vi "getAngle.vi"(6 "Axis":T1, 8 "error in (no error)":errorcluster, 11 "Instrument.Cryostat in":refnum<class "Instrument.Cryostat.lvclass">) -> (0 "error out":errorcluster, 1 "Status":string, 2 "Angle (°)":dbl, 3 "Instrument.Cryostat out":refnum<class "Instrument.Cryostat.lvclass">)   [LabVIEW 2019, in "Instrument.Cryostat.lvclass"]
uses:
  Instrument.Cryostat.lvclass
  C:/Users/patrick/Documents/GitHub/Instrument-Framework/lvsrc/Instrument/Instrument.lvclass
  Typedefs/Rotator Axis--Enum.ctl
  Typedefs/getAngle--cluster.ctl
  Instrument/Instrument.lvclass/Instrument.ctl
  d7de1868-e79d-4787-9e9f-00102efb34a0.vi
  d7de1868-e79d-4787-9e9f-00102efb34a0.vi/29015152-4dd0-45c0-ae7b-e0ee80cdf932.vi
  d7de1868-e79d-4787-9e9f-00102efb34a0.vi/78c8e4cc-1710-4685-8e18-4a9f090162ba.vi
  Instrument/Private/Get Client Type.vi
  d7de1868-e79d-4787-9e9f-00102efb34a0.vi/29015152-4dd0-45c0-ae7b-e0ee80cdf932.vi/49513277-8b05-47b5-8656-0540af669f9a.vi
  d7de1868-e79d-4787-9e9f-00102efb34a0.vi/29015152-4dd0-45c0-ae7b-e0ee80cdf932.vi/bcc89b85-e935-4bd8-847f-6a809bd2d440.vi
  Instrument/Private/Set Dependencies.vi
  d7de1868-e79d-4787-9e9f-00102efb34a0.vi/78c8e4cc-1710-4685-8e18-4a9f090162ba.vi/8cbdd292-283f-4f32-a3cc-82cdd24e7583.vi
  d7de1868-e79d-4787-9e9f-00102efb34a0.vi/78c8e4cc-1710-4685-8e18-4a9f090162ba.vi/036cd682-c314-48e0-a153-600fb577c118.vi
  d7de1868-e79d-4787-9e9f-00102efb34a0.vi/78c8e4cc-1710-4685-8e18-4a9f090162ba.vi/5d11e547-53d6-4100-b73f-5ffdf814e87d.vi
  d7de1868-e79d-4787-9e9f-00102efb34a0.vi/29015152-4dd0-45c0-ae7b-e0ee80cdf932.vi/bcc89b85-e935-4bd8-847f-6a809bd2d440.vi/2e8ce9c0-d7f6-46c2-b56a-ccad562160a9.vi
  d7de1868-e79d-4787-9e9f-00102efb34a0.vi/29015152-4dd0-45c0-ae7b-e0ee80cdf932.vi/bcc89b85-e935-4bd8-847f-6a809bd2d440.vi/071ed579-4f01-4414-bbcb-77796d1fffd3.vi
  d7de1868-e79d-4787-9e9f-00102efb34a0.vi/78c8e4cc-1710-4685-8e18-4a9f090162ba.vi/036cd682-c314-48e0-a153-600fb577c118.vi/f30586f2-7be0-47a0-9240-ffa99525c1ce.vi
  d7de1868-e79d-4787-9e9f-00102efb34a0.vi/78c8e4cc-1710-4685-8e18-4a9f090162ba.vi/036cd682-c314-48e0-a153-600fb577c118.vi/7bb9839c-ec85-4b4c-931f-28db1f4f848b.vi
  d7de1868-e79d-4787-9e9f-00102efb34a0.vi/78c8e4cc-1710-4685-8e18-4a9f090162ba.vi/5d11e547-53d6-4100-b73f-5ffdf814e87d.vi/70780e69-106e-4e28-be9f-45ae0745826c.vi
  d7de1868-e79d-4787-9e9f-00102efb34a0.vi/78c8e4cc-1710-4685-8e18-4a9f090162ba.vi/5d11e547-53d6-4100-b73f-5ffdf814e87d.vi/f098dfd7-b95c-4643-8807-c1855e54edfe.vi
  Instrument/Private/Get RC Connection Status.vi
  Instrument/Private/Get Dependencies.vi
  <userlib>/LevyLab/RemoteControl/API/Send and Receive.vi
  <vilib>/Utility/Data Type/Get Type Information.vi
  <vilib>/JDP Science/JSONtext/JSON text to Variant.vi
  Instrument/API/Instrument.GetPublicEvents.vi
  <vilib>/JDP Science/JSONtext/Variant to JSON Text.vi
  <vilib>/National Instruments/GUID Generator/Guid Generator.vi
  Instrument/API/Instrument.sendMessageToProcess.vi
  Instrument/Private/Instrument.MessageFromProcess.EventStructure.vi
  <vilib>/JDP Science/JSONtext/LVClass Serializer/JSONtext LVClass Serializer.lvclass
  Instrument/Instrument.lvclass
panel:
  out "Finished?":bool
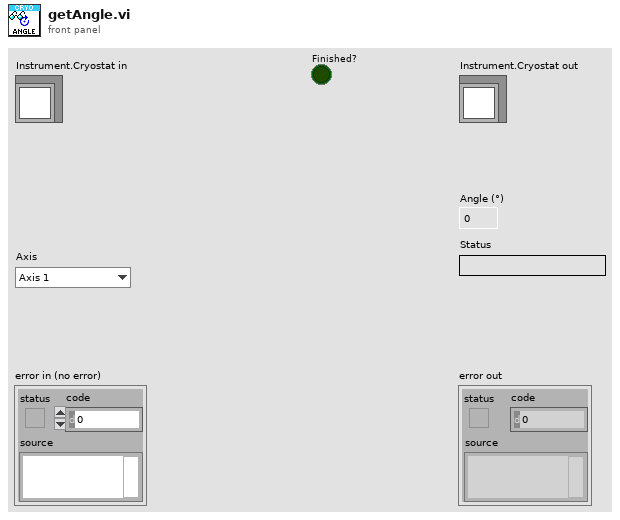
[diagram p1: front panel]
types:
  T1 = typedef "Instrument.Cryostat.lvclass/Rotator Axis--Enum.ctl" = enum16{"Axis 1", "Axis 2"}
  T2 = typedef "Instrument.Cryostat.lvclass/getAngle--cluster.ctl" = cluster{"Angle":dbl, "Status":string, "Finished?":bool}
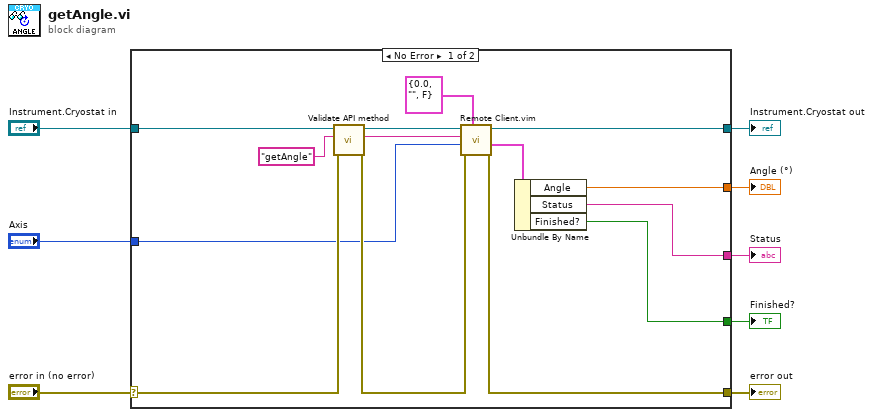
[diagram p0: block diagram]
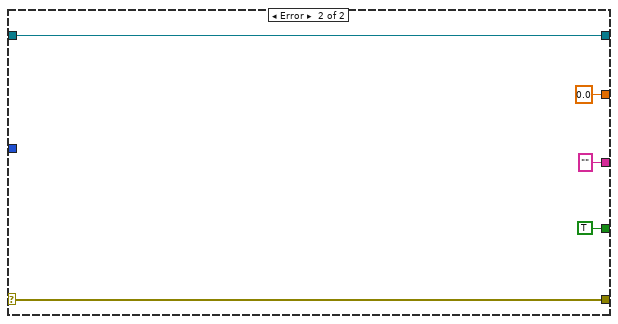
[diagram p2: hidden frame]
diagram:
  n1 = case shown="No Error" "error in (no error)" {
    selector: "error in (no error)" -> [w16 w27]
    tunnel: [w14 w27] -> w7
    tunnel: [w17 w26] -> w5
    tunnel: "Instrument.Cryostat in" -> [w18 w26]
    tunnel: "Axis" -> [w13 _]
    tunnel: [w11 0.0 ("Angle (°)")] -> w3
    tunnel: [w10 "" ("Status")] -> w2
    tunnel: [w9 TRUE ("Finished?")] -> w1
    frame No Error {
      n2 = call "Validate API method.vi"("error in (no error)"=w16, "command in"="getAngle" ("error message (\"\")"), "Instrument in"=w18) -> ("error out"=w15:errorcluster, "command out"=w21:string, "Instrument out"=w20:refnum<class "Instrument.Cryostat.lvclass">)  [unwired: 6 in]
      n3 = call "Remote Client.vim"("Data Out type"=T2 {"Angle"=0.0, "Status"="", "Finished?"=FALSE} ("getAngle"), "error in (no error)"=w15, "params"=w13, "method"=w21, "Instrument in"=w20) -> ("error out"=w14:errorcluster, "Data out"=w19:T2, "Instrument out"=w17:refnum<class "Instrument.Cryostat.lvclass">)  [unwired: 3 in, 1 out]
      n4 = Unbundle By Name(w19) -> ("Angle"=w11:dbl, "Status"=w10:string, "Finished?"=w9:bool)
    }
    frame Error {
    }
  }
  "error out" <- w7
  "Instrument.Cryostat out" <- w5
  "Angle (°)" <- w3
  "Status" <- w2
  "Finished?" <- w1
